vi "Test Error Message.vi"() -> ()   [LabVIEW 2012]
panel:
  in  "Boolean":bool
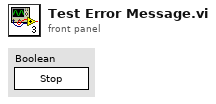
[diagram p1: front panel]
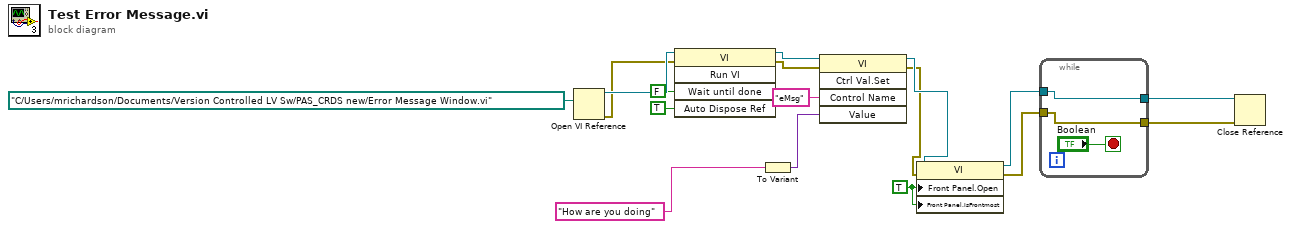
[diagram p0: block diagram]
diagram:
  w4 = TRUE ("Front Panel Window:Open")
  n1 = Open VI Reference(vi path=path "C:/Users/mrichardson/Documents/Version Controlled LV Sw/PAS_CRDS new/Error Message Window.vi") -> (vi reference=w16:refnum<vi>, error out=w8:errorcluster)  [unwired: 5 in]
  n2 = invoke class="VI" method="Run VI"(reference=w16, error in=w8, "Wait until done"=FALSE ("Wait Until Done"), "Auto Dispose Ref"=TRUE ("Auto Dispose Reference")) -> (reference out=w15:refnum<vi>, error out=w9:errorcluster)  [unwired: 1 in, 3 out]
  n3 = To Variant(anything="How are you doing" ("Control Name")) -> (Variant=w12:variant)
  n4 = invoke class="VI" method="Ctrl Val.Set"(reference=w15, error in=w9, "Control Name"="eMsg", "Value"=w12) -> (reference out=w5:refnum<vi>, error out=w3:errorcluster)  [unwired: 1 in, 3 out]
  n5 = property class="VI"(reference=w5, error in=w3, "Front Panel.Open"=w4, "Front Panel.IsFrontmost"=w4) -> (reference out=w2:refnum<vi>, error out=w1:errorcluster)
  n6 = while {
    tunnel: w2 -> [w19]
    tunnel: w1 -> [w18]
    tunnel: [w19] -> w11
    tunnel: [w18] -> w10
    stop <- "Boolean" stop-if-true
  }
  n7 = Close Reference(reference=w11, error in (no error)=w10) -> ()  [unwired: 1 out]
